vi "Actor Core.vi"(8 "error in":errorcluster, 11 "Nested in":refnum<class "[MV] Key Generator.lvclass">) -> (0 "error out":errorcluster, 3 "Actor out":refnum<class "Actor.lvclass">)   [LabVIEW 2023, in "[MV] Key Generator.lvlib" / "[MV] Key Generator.lvclass"]
doc: "(<B>Filename</B>: Actor Framework.lvlib:Actor.lvclass:Actor Core.vi)\n\nReceives messages to the actor, reacts to them, and initiates any error handling that may shut the actor down.\n\nDescendant classes may override this VI to append parallel tasks for the actor to complete while it handles messages. Overrides use the Call Parent Method node."
uses:
  [MV] Key Generator.lvclass
  C:/Program Files (x86)/National Instruments/LabVIEW 2023/vi.lib/ActorFramework/Actor/Actor.lvclass
  <vilib>/ActorFramework/Actor/Actor.lvclass
  <vilib>/ActorFramework/Actor/Actor.lvclass/Actor.ctl
  <vilib>/ActorFramework/Message Enqueuer/Message Enqueuer.lvclass/Message Enqueuer.ctl
  [MV] Key Generator.lvclass/[MV] Key Generator.ctl
  <vilib>/ActorFramework/Message Enqueuer/Init from Existing Queue.vi
  <vilib>/ActorFramework/Message Enqueuer/Enqueue.vi
  [MV] Key Generator Messages/Event New SW Msg/Event New SW Msg.lvclass
  C:/Program Files (x86)/National Instruments/LabVIEW 2023/vi.lib/ActorFramework/Message/Message.lvclass
  [MV] Key Generator Messages/Event Delete SW Msg/Event Delete SW Msg.lvclass
  [MV] Key Generator Messages/Event Keygen Msg/Event Keygen Msg.lvclass
  [MV] Key Generator Messages/Event Software Msg/Event Software Msg.lvclass
  <vilib>/ActorFramework/Stop Msg/Stop Msg.lvclass
  <vilib>/ActorFramework/Message Priority Queue/Priority Enqueue.vi
  <vilib>/ActorFramework/Message Enqueuer/Message Enqueuer.lvclass
panel:
  out "public key":string caption="公钥"
  in  "delete sw":bool caption="new software"
  in  "new sw":bool caption="new software"
  in  "keygen":bool caption="generate"
  out "key":string caption="激活码"
  in  "machine code":string caption="机器码"
  in  "valid time":i16(ring)=7 caption="有效时间" items=["7天"=7, "30天"=30, "90天"=90, "永久"=-1]
  in  "software":u16(ring) caption="软件名称"
  # "注 册 机"
  # "1. 选择或创建软件；\n2. 选择激活码有效时间；\n3. 粘贴机器码；\n4. 点击 “生成激活码” 按钮；\n5. 复制激活码。"
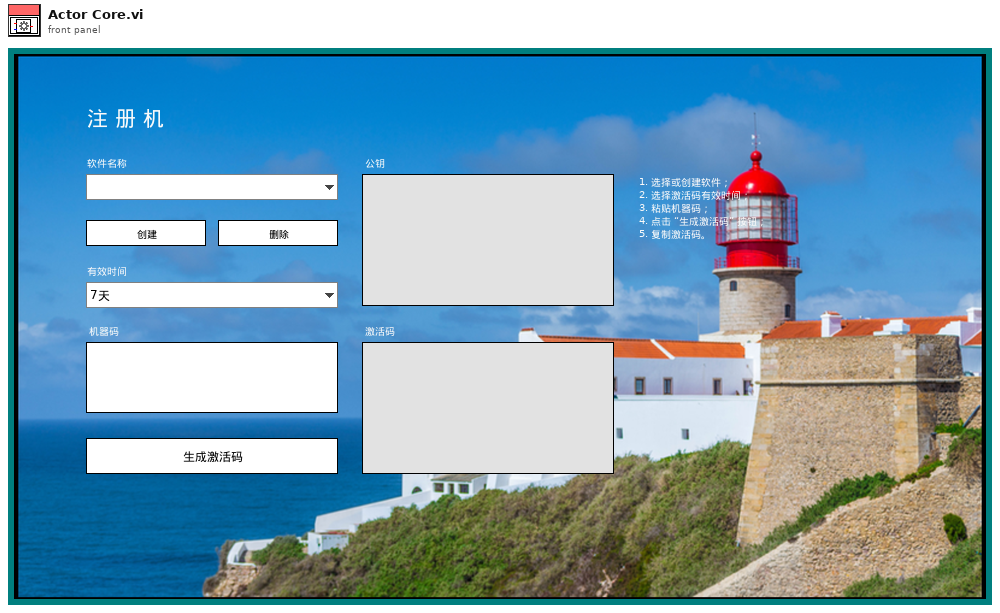
[diagram p1: front panel]
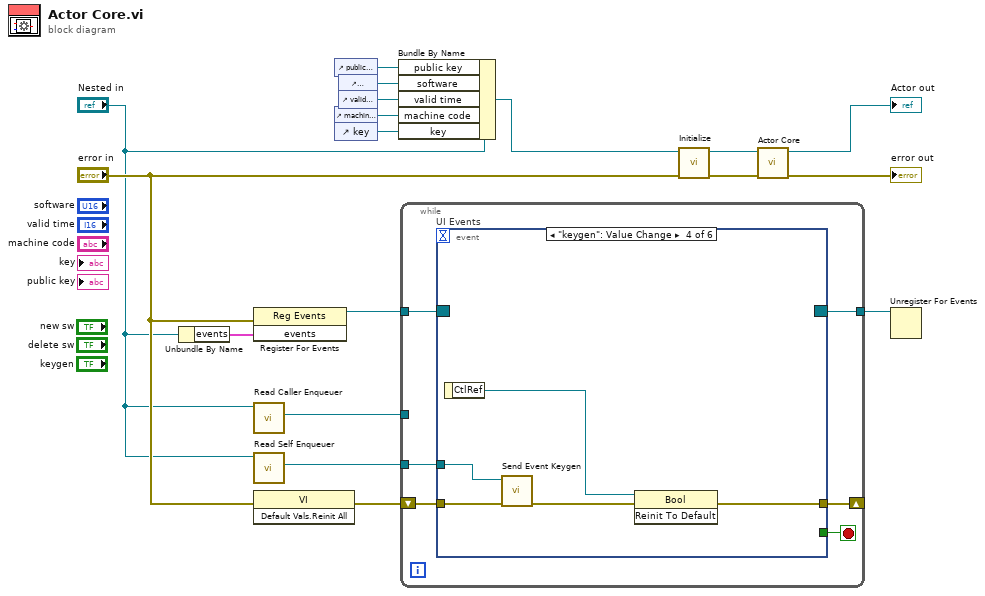
[diagram p0: block diagram]
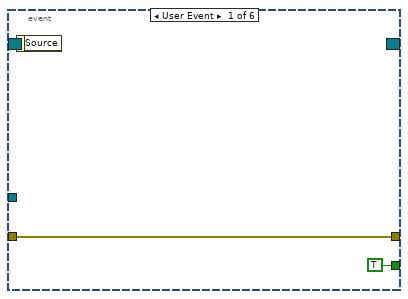
[diagram p2: hidden frame]
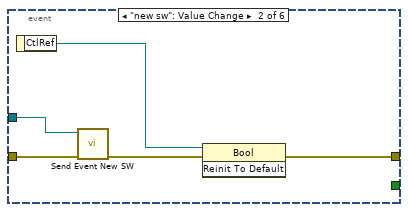
[diagram p3: hidden frame]
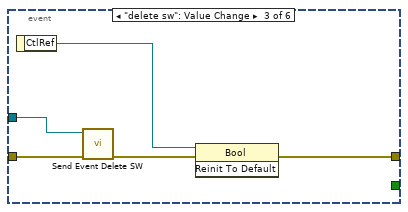
[diagram p4: hidden frame]
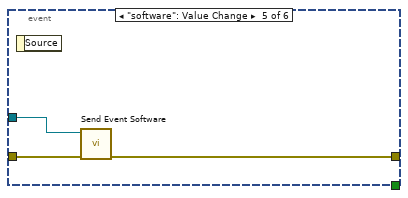
[diagram p5: hidden frame]
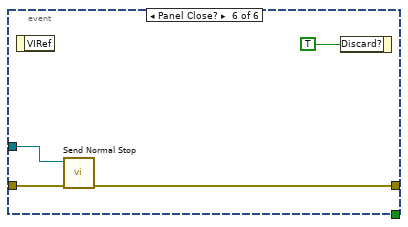
[diagram p6: hidden frame]
diagram:
  n1 = Unbundle By Name("Nested in") -> ("events"=w15:cluster{"stop":refnum<user-event>})
  n2 = register-events ("Main Register for Events")(error in="error in", w15) -> (reference out=w16:refnum<event-registration>)  [unwired: 1 in, 1 out]
  n3 = call <vilib>:"Read Caller Enqueuer.vi"("Actor"="Nested in") -> ("Caller Enqueuer"=w12:refnum<class "Message Enqueuer.lvclass">)  [unwired: 10 in]
  n4 = call <vilib>:"Read Self Enqueuer.vi"("Actor"="Nested in") -> ("Self Enqueuer"=w13:refnum<class "Message Enqueuer.lvclass">)  [unwired: 10 in]
  n5 = invoke class="VI" method="Default Vals.Reinit All"(error in="error in") -> (error out=w11:errorcluster)  [unwired: 2 in, 2 out]
  n6 = control-ref of="public key"() -> (w1:refnum<vi>)
  n7 = control-ref of="machine code"() -> (w3:refnum<vi>)
  n8 = control-ref of="key"() -> (w2:refnum<vi>)
  n9 = control-ref of="software"() -> (w5:refnum<vi>)
  n10 = control-ref of="valid time"() -> (w4:refnum<vi>)
  n11 = Bundle By Name(cluster="Nested in", "public key"=w1, "software"=w5, "valid time"=w4, "machine code"=w3, "key"=w2) -> (w6:refnum<class "[MV] Key Generator.lvclass">)
  n12 = while {
    tunnel: w16 -> [w24]
    tunnel: [w22] -> w14
    tunnel: w13 -> [w21]
    tunnel: w12 -> [_]
    shift-right: [w19] -> _
    shift-left: w11 -> [w20]
    stop <- w23 stop-if-true
    n13 = event "UI Events" shown="[3] \"keygen\": Value Change" {
      selector: w24 -> [_ _ _ _ _ _]
      dyn-events: [_ _ _ _ _ _] -> w22
      timeout: _ -> [_ _ _ _ _ _]
      tunnel: [TRUE _ _ _ _ _] -> w23
      tunnel: w21 -> [_ w30 w35 w40 w43 w47]
      tunnel: w20 -> [w26 w31 w36 w41 w44 w46]
      tunnel: [w26 w27 w33 w37 w42 w45] -> w19
      event User Event {
        n14 = event-data() -> ()  [unwired: 1 in, 1 out]
      }
      event "new sw": Value Change {
        n15 = event-data() -> ("CtlRef"=w28:refnum<vi>)  [unwired: 1 in]
        n16 = call "Send Event New SW.vi"("error in (no error)"=w31, "Message Enqueuer"=w30) -> ("error out"=w29:errorcluster)  [unwired: 8 in, 1 out]
        n17 = invoke class="Bool" method="Reinit To Default"(reference=w28, error in=w29) -> (error out=w27:errorcluster)  [unwired: 1 in, 2 out]
      }
      event "delete sw": Value Change {
        n18 = event-data() -> ("CtlRef"=w32:refnum<vi>)  [unwired: 1 in]
        n19 = call "Send Event Delete SW.vi"("error in (no error)"=w36, "Message Enqueuer"=w35) -> ("error out"=w34:errorcluster)  [unwired: 8 in, 1 out]
        n20 = invoke class="Bool" method="Reinit To Default"(reference=w32, error in=w34) -> (error out=w33:errorcluster)  [unwired: 1 in, 2 out]
      }
      event "keygen": Value Change {
        n21 = event-data() -> ("CtlRef"=w38:refnum<vi>)  [unwired: 1 in]
        n22 = call "Send Event Keygen.vi"("error in (no error)"=w41, "Message Enqueuer"=w40) -> ("error out"=w39:errorcluster)  [unwired: 8 in, 1 out]
        n23 = invoke class="Bool" method="Reinit To Default"(reference=w38, error in=w39) -> (error out=w37:errorcluster)  [unwired: 1 in, 2 out]
      }
      event "software": Value Change {
        n24 = event-data() -> ()  [unwired: 1 in, 1 out]
        n25 = call "Send Event Software.vi"("error in (no error)"=w44, "Message Enqueuer"=w43) -> ("error out"=w42:errorcluster)  [unwired: 8 in, 1 out]
      }
      event Panel Close? {
        n26 = event-data() -> ()  [unwired: 1 in, 1 out]
        n27 = call <vilib>:"Send Normal Stop.vi"("error in (no error)"=w46, "Message Enqueuer"=w47) -> ("error out"=w45:errorcluster)  [unwired: 9 in]
        n28 = event-data("Discard?"=TRUE) -> ()  [unwired: 1 in, 1 out]
      }
    }
  }
  n29 = call "Initialize.vi"("error in (no error)"="error in", "View Template in"=w6) -> ("error out"=w10:errorcluster, "View Template out"=w9:refnum<class "[MV] Key Generator.lvclass">)  [unwired: 8 in]
  n30 = call-parent "Actor Core.vi"("error in"=w10, "Actor in"=w9) -> ("error out"=→"error out":errorcluster, "Actor out"=→"Actor out":refnum<class "Actor.lvclass">)  [unwired: 8 in]
  n31 = Unregister For Events(event registration refnum=w14) -> ()  [unwired: 1 in, 1 out]
